vi "Globals.vi"() -> ()   [LabVIEW 2019, in "RT_Game.lvlib" / "Engine.lvclass"]
uses:
  Engine.lvclass
panel:
  out "Stop?":bool
  out "CameraMoving?":bool
  in  "volume_effects":dbl=0.2
  in  "volume_music":dbl=0.2
  in  "deltaT":dbl
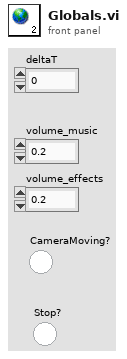
[diagram p1: front panel]
diagram:
